vi "VISATCP组合选择发送.vi"(0 "IP":string, 1 "数据发送通道":enum16{"TCP", "VISA"}(ring), 2 "命令":string(combo), 5 "PORT":string, 7 "VISA resource name":refnum<visa-resource-name> caption="VISA资源名称", 9 "baud rate":u32=115200 caption="波特率(115200)", 11 "error in (no error)":errorcluster caption="错误输入（无错误）", 12 "写入缓冲区":string) -> (4 "连接ID":refnum<k5>, 6 "VISA resource name 2":refnum<visa-resource-name>, 13 "读取缓冲区":string, 15 "错误输出":errorcluster)   [LabVIEW 2016, in "数据传输系统-05.lvlib"]
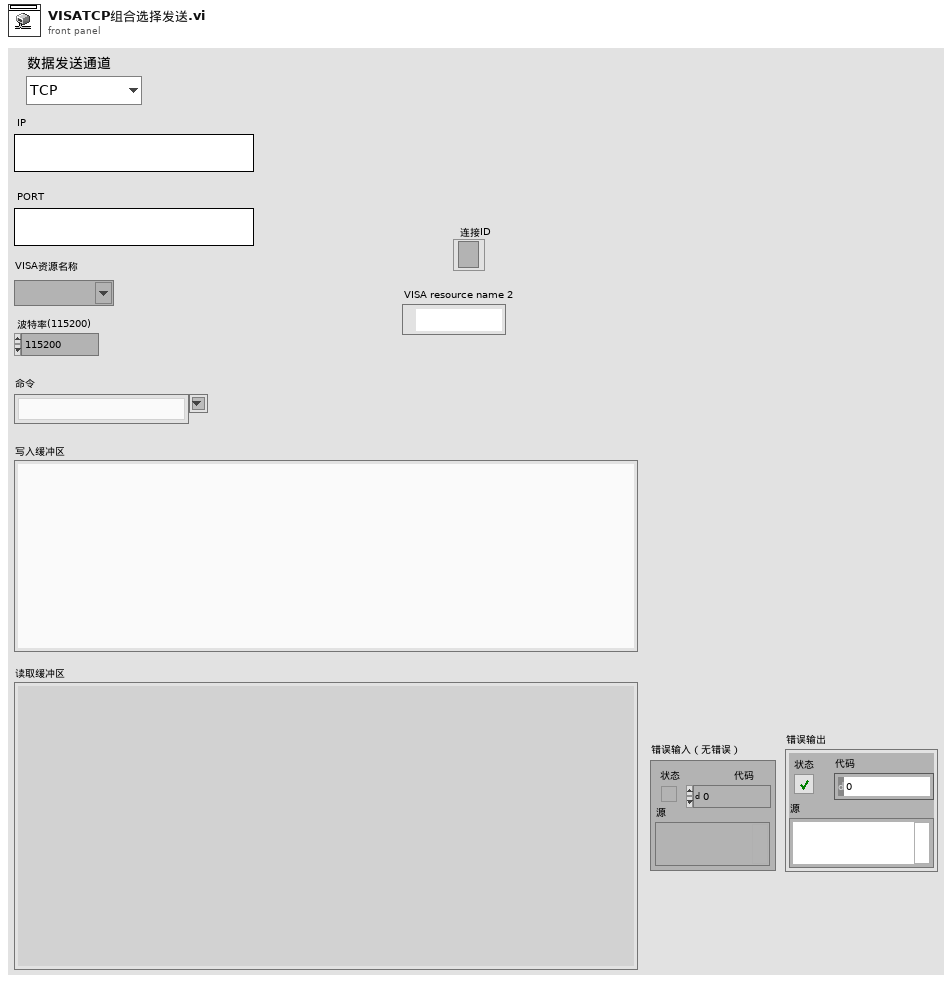
[diagram p1: front panel]
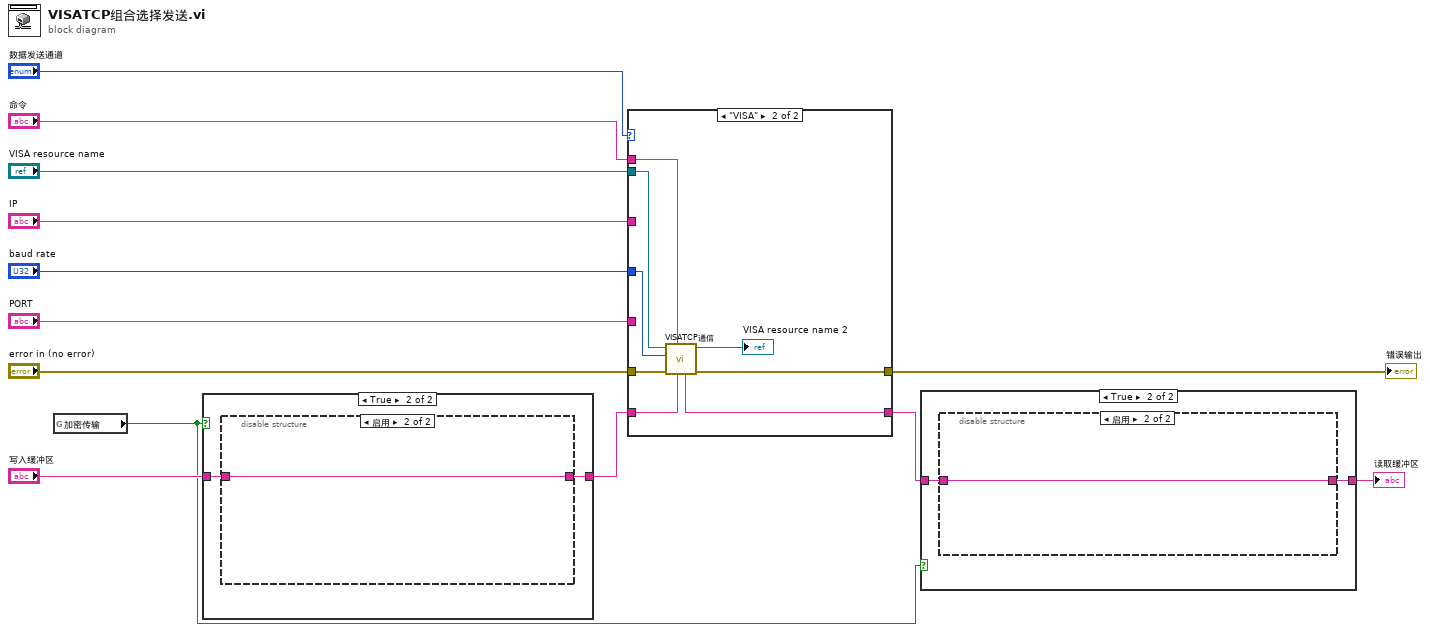
[diagram p0: block diagram]
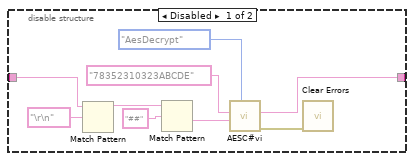
[diagram p3: hidden frame]
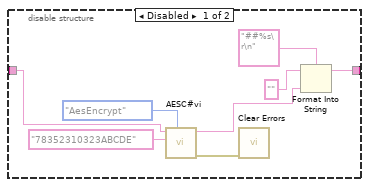
[diagram p5: hidden frame]
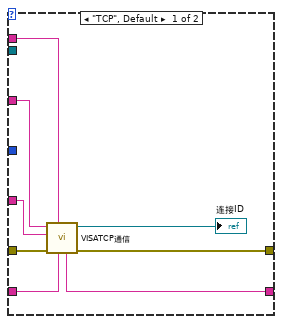
[diagram p6: hidden frame]
diagram:
  n1 = global read "断电保存全局.vi" "加密传输"() -> (w3:bool)
  n2 = case shown="True" w3 {
    tunnel: "写入缓冲区" -> [w14 w16]
    tunnel: [w14 w15] -> w4
    frame False {
    }
    frame True {
      n3 = disable-structure shown="启用" {
        disable-tunnel: w16 -> [w19 w25]
        disable-tunnel: [w18 w25] -> w15
        frame Disabled {
          n4 = call "AESC#vi.vi"("枚举"=enum16{"AesEncrypt", "AesDecrypt"}."AesEncrypt", "key"="78352310323ABCDE", "plainText"=w19) -> ("错误输出"=w17:errorcluster, "AESEncrypt"=w20:string)  [unwired: 6 in, 1 out]
          n5 = call <vilib>:"Clear Errors.vi"("error in (no error)"=w17) -> ()  [unwired: 5 in, 2 out]
          n6 = Format Into String(format string="##%s\r\n", initial string="" ("初始字符串"), w20) -> (resulting string=w18:string)  [unwired: 1 in, 1 out]
        }
        frame Enabled {
        }
      }
    }
  }
  n7 = case shown="\"VISA\"" "数据发送通道" {
    tunnel: "命令" -> [w33 w37]
    tunnel: [w32 w39] -> w11
    tunnel: "error in (no error)" -> [w31 w38]
    tunnel: w4 -> [w30 w41]
    tunnel: [w29 w40] -> w2
    tunnel: "PORT" -> [w28 _]
    tunnel: "IP" -> [w27 _]
    tunnel: "baud rate" -> [_ w35]
    tunnel: "VISA resource name" -> [_ w34]
    frame "TCP", Default {
      n8 = call-poly "VISATCP通信.vi"("写入缓冲区"=w30, "命令"=w33, "error in (no error)"=w31, "PORT"=w28, "IP"=w27) -> ("错误输出"=w32:errorcluster, "连接ID"=→"连接ID":refnum<k5>, "读取缓冲区"=w29:string)  [unwired: 4 in]
    }
    frame "VISA" {
      n9 = call-poly "VISATCP通信.vi"("写入缓冲区"=w41, "命令"=w37, "error in (no error)"=w38, "baud rate (9600)"=w35, "VISA resource name"=w34) -> ("错误输出"=w39:errorcluster, "VISA resource name 2"=→"VISA resource name 2":refnum<visa-resource-name>, "读取缓冲区"=w40:string)  [unwired: 4 in]
    }
  }
  "错误输出" <- w11
  n10 = case shown="True" w3 {
    tunnel: w2 -> [w42 w43]
    tunnel: [w42 w44] -> w1
    frame False {
    }
    frame True {
      n11 = disable-structure shown="启用" {
        disable-tunnel: [w49 w54] -> w44
        disable-tunnel: w43 -> [w47 w54]
        frame Disabled {
          n12 = Match Pattern(string=w47, regular expression="\r\n" ("正则表达式")) -> (before substring=w46:string)  [unwired: 1 in, 3 out]
          n13 = Match Pattern(string=w46, regular expression="##" ("正则表达式")) -> (after substring=w45:string)  [unwired: 1 in, 3 out]
          n14 = call "AESC#vi.vi"("枚举"=enum16{"AesEncrypt", "AesDecrypt"}."AesDecrypt", "encryptStr"=w45, "key"="78352310323ABCDE") -> ("错误输出"=w48:errorcluster, "AESDecrypt"=w49:string)  [unwired: 6 in, 1 out]
          n15 = call <vilib>:"Clear Errors.vi"("error in (no error)"=w48) -> ()  [unwired: 5 in, 2 out]
        }
        frame Enabled {
        }
      }
    }
  }
  "读取缓冲区" <- w1
